vi "Destroy Sync Refnums.vi"(8 "error in":errorcluster, 9 "Module ID":i32) -> (0 "error out":errorcluster)   [LabVIEW 2024, in "cameraV1.lvlib"]
doc: "Destroy the sync refnums used to synchronize event generation, event registration and stop module between the module and its caller(s).\n_____\nBased on DQMH Dev Tools: Project Template 7.1.0.1503."
uses:
  cameraV1.lvlib
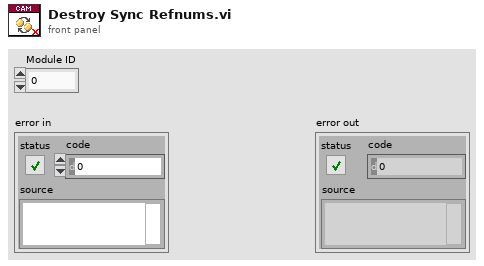
[diagram p1: front panel]
types:
  T1 = typedef "Rendezvous RefNum" = refnum<k1>
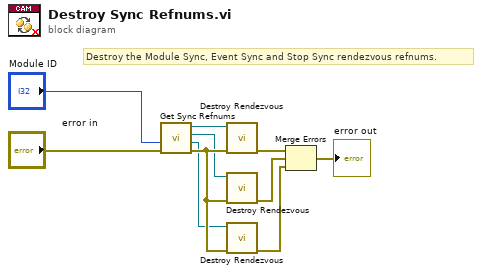
[diagram p0: block diagram]
diagram:
  # "Destroy the Module Sync, Event Sync and Stop Sync rendezvous refnums."
  n1 = call "Get Sync Refnums.vi"("error in"="error in", "Module ID"="Module ID") -> ("error out"=w10:errorcluster, "Stop Sync"=w2:T1, "Event Sync"=w6:T1, "Module Sync"=w8:T1)  [unwired: 6 in]
  n2 = call <vilib>:"Destroy Rendezvous.vi"("error in (no error)"=w10, "rendezvous"=w8) -> ("error out"=w7:errorcluster)  [unwired: 4 in, 1 out]
  n3 = call <vilib>:"Destroy Rendezvous.vi"("error in (no error)"=w10, "rendezvous"=w6) -> ("error out"=w4:errorcluster)  [unwired: 4 in, 1 out]
  n4 = call <vilib>:"Destroy Rendezvous.vi"("error in (no error)"=w10, "rendezvous"=w2) -> ("error out"=w1:errorcluster)  [unwired: 4 in, 1 out]
  n5 = Merge Errors(w7, w4, w1) -> (→"error out":errorcluster)
